vi "FalconSwerveVelocityConversion.vi"(1 "Velocity (Raw Sensor Units per 100 ms)":i32) -> (0 "Velocity (ft/s)":dbl)   [LabVIEW 2020]
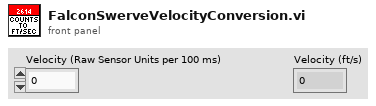
[diagram p1: front panel]
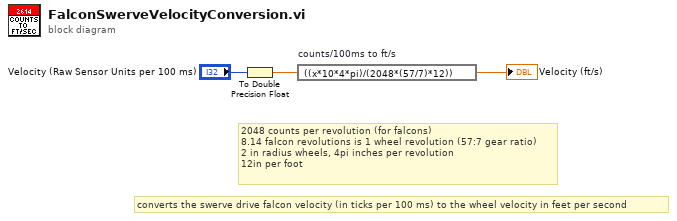
[diagram p0: block diagram]
diagram:
  # "converts the swerve drive falcon velocity (in ticks per 100 ms) to the wheel velocity in feet per second"
  # "2048 counts per revolution (for falcons)\n8.14 falcon revolutions is 1 wheel revolution (57:7 gear ratio)\n2 in radius wheels, 4pi inches per revolution\n12in per foot"
  n1 = To Double Precision Float(number="Velocity (Raw Sensor Units per 100 ms)") -> (double precision float=w2:dbl)
  n2 = expression code="((x*10*4*pi)/(2048*(57/7)*12))" "counts/100ms to ft/s"(w2) -> (→"Velocity (ft/s)":dbl)
